vi "PS.vi"(9 "Imaginary In":fxp<+/-,64,32>[](array[numeric]), 10 "Real In":fxp<+/-,64,32>[](array[numeric])) -> (2 "Power Spectrum":fxp<+/-,64,32>[](array[numeric]))   [LabVIEW 2015]
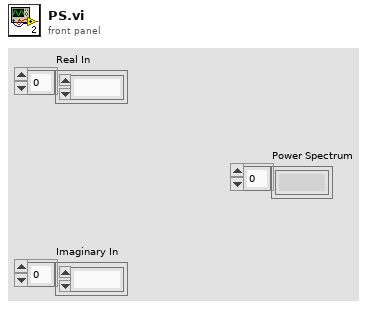
[diagram p1: front panel]
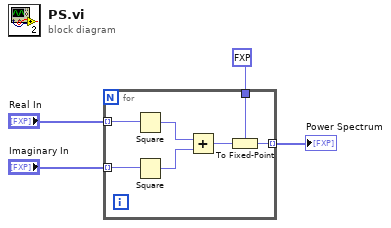
[diagram p0: block diagram]
diagram:
  n1 = for {
    tunnel: [w9] -> w1 mode=indexing
    tunnel: "Real In" -> [w7] mode=indexing
    tunnel: "Imaginary In" -> [w8] mode=indexing
    tunnel: fxp<+/-,64,32> 0.0 ("Real In") -> [w10]
    n2 = Square(x=w7) -> (x^2=w6:fxp<+,64,63>)
    n3 = Square(x=w8) -> (x^2=w5:fxp<+,64,63>)
    n4 = Add(x=w6, y=w5) -> (x+y=w11:fxp<+,64,64>)
    n5 = To Fixed-Point(fixed-point type=w10, number=w11) -> (fixed-point=w9:fxp<+/-,64,32>)
  }
  "Power Spectrum" <- w1
